vi "Encoder Init.vi"(8 "error in (no error)":errorcluster) -> (0 "error out":errorcluster, 3 "TitanENC out":T1)   [LabVIEW 2020]
uses:
  <vilib>/High Genius/HG_WSI_Tookit/Dependencies/Library/TitanENC/TitanENC.lvclass
  C:/Program Files (x86)/National Instruments/LabVIEW 2020/vi.lib/High Genius/HG_WSI_Tookit/Dependencies/Library/HG_LIB/HG_LIB.lvclass
  <vilib>/High Genius/HG_WSI_Tookit/Dependencies/Library/HG_LIB/HG_LIB.lvclass
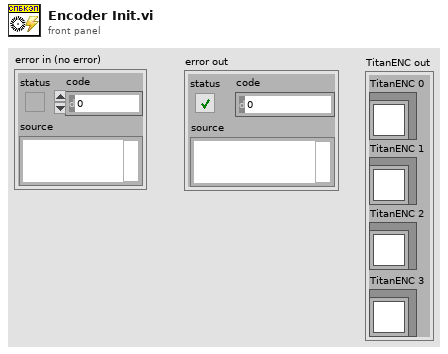
[diagram p1: front panel]
types:
  T1 = cluster{"TitanENC 0":refnum<class "TitanENC.lvclass">, "TitanENC 1":refnum<class "TitanENC.lvclass">, "TitanENC 2":refnum<class "TitanENC.lvclass">, "TitanENC 3":refnum<class "TitanENC.lvclass">}
  T2 = enum16{"0", "1", "2", "3", "4", "5", "6", "7", "8", "9", "10", "11", "12", "13", "14", "15", "16", "17", "18", "19", "20", "21", "22", "23", "24", "25"}
  T3 = enum16{"DI", "DO", "AI", "Pulse", "PWM", "ISQ", "ENC", "CAN", "IIC", "IMU"}
  T4 = cluster{"HG_LIB out":refnum<class "TitanENC.lvclass">, "HG_LIB out":refnum<class "TitanENC.lvclass">, "HG_LIB out":refnum<class "TitanENC.lvclass">, "HG_LIB out":refnum<class "TitanENC.lvclass">}
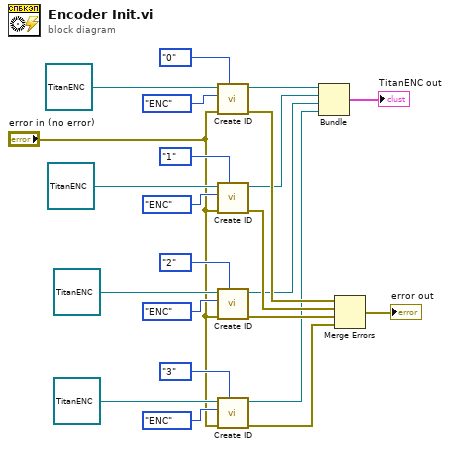
[diagram p0: block diagram]
diagram:
  n1 = call <vilib>:"Create ID.vi"("NO"=T2."0", "error in (no error)"="error in (no error)", "Function"=T3."ENC", "HG_LIB in"=refnum<class "TitanENC.lvclass"> refnum ("VMX Library.lvlib:TitanENC.lvclass")) -> ("error out"=w12:errorcluster, "HG_LIB out"=w11:refnum<class "TitanENC.lvclass">)  [unwired: 6 in]
  n2 = call <vilib>:"Create ID.vi"("NO"=T2."1", "error in (no error)"="error in (no error)", "Function"=T3."ENC", "HG_LIB in"=refnum<class "TitanENC.lvclass"> refnum ("VMX Library.lvlib:TitanENC.lvclass")) -> ("error out"=w13:errorcluster, "HG_LIB out"=w10:refnum<class "TitanENC.lvclass">)  [unwired: 6 in]
  n3 = call <vilib>:"Create ID.vi"("NO"=T2."2", "error in (no error)"="error in (no error)", "Function"=T3."ENC", "HG_LIB in"=refnum<class "TitanENC.lvclass"> refnum ("VMX Library.lvlib:TitanENC.lvclass")) -> ("error out"=w14:errorcluster, "HG_LIB out"=w9:refnum<class "TitanENC.lvclass">)  [unwired: 6 in]
  n4 = call <vilib>:"Create ID.vi"("NO"=T2."3", "error in (no error)"="error in (no error)", "Function"=T3."ENC", "HG_LIB in"=refnum<class "TitanENC.lvclass"> refnum ("VMX Library.lvlib:TitanENC.lvclass")) -> ("error out"=w1:errorcluster, "HG_LIB out"=w2:refnum<class "TitanENC.lvclass">)  [unwired: 6 in]
  n5 = Bundle("HG_LIB out"=w11, "HG_LIB out"=w10, "HG_LIB out"=w9, "HG_LIB out"=w2) -> (→"TitanENC out":T4)  [unwired: 1 in]
  n6 = Merge Errors(w12, w13, w14, w1) -> (→"error out":errorcluster)
